vi "read_wav_to_data_fpga tester.vi"() -> ()   [LabVIEW 2021]
uses:
  <vilib>/rvi/interface/nirviOpenFPGA/nirviOpenFPGA.xnode
  <vilib>/rvi/interface/nirviReadWriteControl/nirviReadWriteControl.xnode
  <vilib>/rvi/interface/nirviMethod/nirviMethod.xnode
  <vilib>/FPGAPlugInAG/Dynamic/niLvFpga_WriteFifo_Dynamic.vi
  <vilib>/rvi/errors/niLvFpgaMergeErrorWithErrorCode.vi
  <vilib>/FPGAPlugInAG/Dynamic/niLvFpga_ReadFifo_Dynamic.vi
  <vilib>/rvi/interface/nirviCloseFPGA/nirviCloseFPGA.xnode
  <instrlib>/_niInstr/Basic Elements/v1/FPGA/niInstr Basic Elements v1 FPGA.lvlib
  <instrlib>/_niInstr/Basic Elements/v1/FPGA/Private/Count Up U16.vi
  FPGA Bitfiles/niUsrpRio200_XcvrTime.lvbitx
  chaim_vis/chaim_Tx.vi
  <vilib>/FPGAPlugInAG/USRP 294xR; 295xR 200 MSps/niLvFpga_Open_USRP 294xR; 295xR 200 MSps.vi
  <vilib>/rvi/interface/common/dynamic/niFpgaDynamicAddResources.vi
  <vilib>/FPGAPlugInAG/Dynamic/niLvFpga_ConfigureFifo_Dynamic.vi
  <vilib>/FPGAPlugInAG/Dynamic/niLvFpga_Close_Dynamic.vi
  NiFpgaLv.dll
  <vilib>/Utility/error.llb/Error Cluster From Error Code.vi
  <vilib>/rvi/interface/Simulation/niFpgaSimulationCallBeginRW.vi
  <vilib>/rvi/errors/niLvFpgaAdjustHostInterfaceError.vi
panel:
  out "Empty Elements Remaining":u32
  out "size(s)":i32
  out "wav sent out":u16
  in  "stop":bool
  in  "millisecond multiple":u32
  out "Waveform Graph 2":dbl[](graph)
  out "error out":errorcluster
  out "UP SAMPLE RATE":fxp<+,48,1>
  out "Numeric":i32
  out "Init Data Out":fxp<+/-,16,1>[](array[numeric])
  out "up sample":dbl format="%#_6f"
  out "attributes":variant
  out "Y 2":dbl[](array[numeric])
  out "dt":dbl format="%#_6p"
  out "t0":timestamp
  out "Y":dbl[](array[numeric])
  out "Waveform Graph":waveform(dbl)[](graph)
  in  "path":path
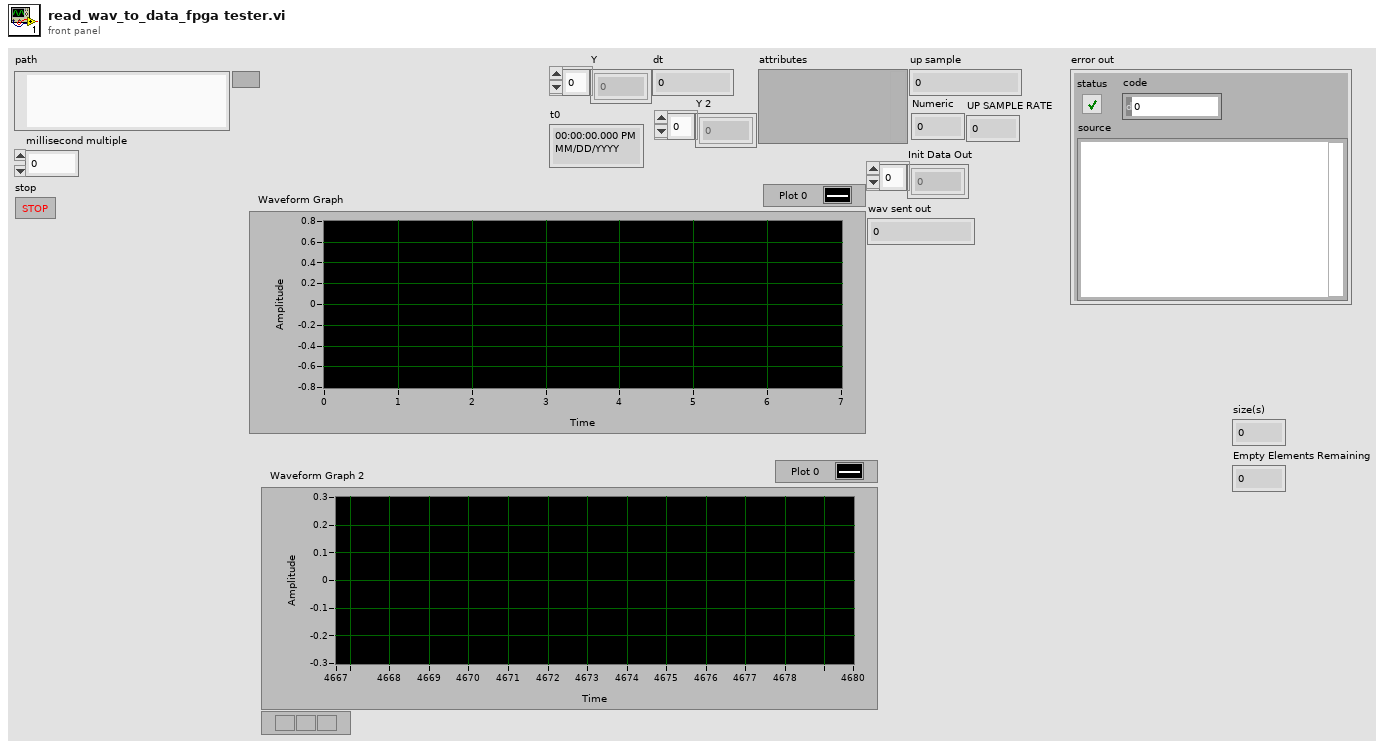
[diagram p1: front panel]
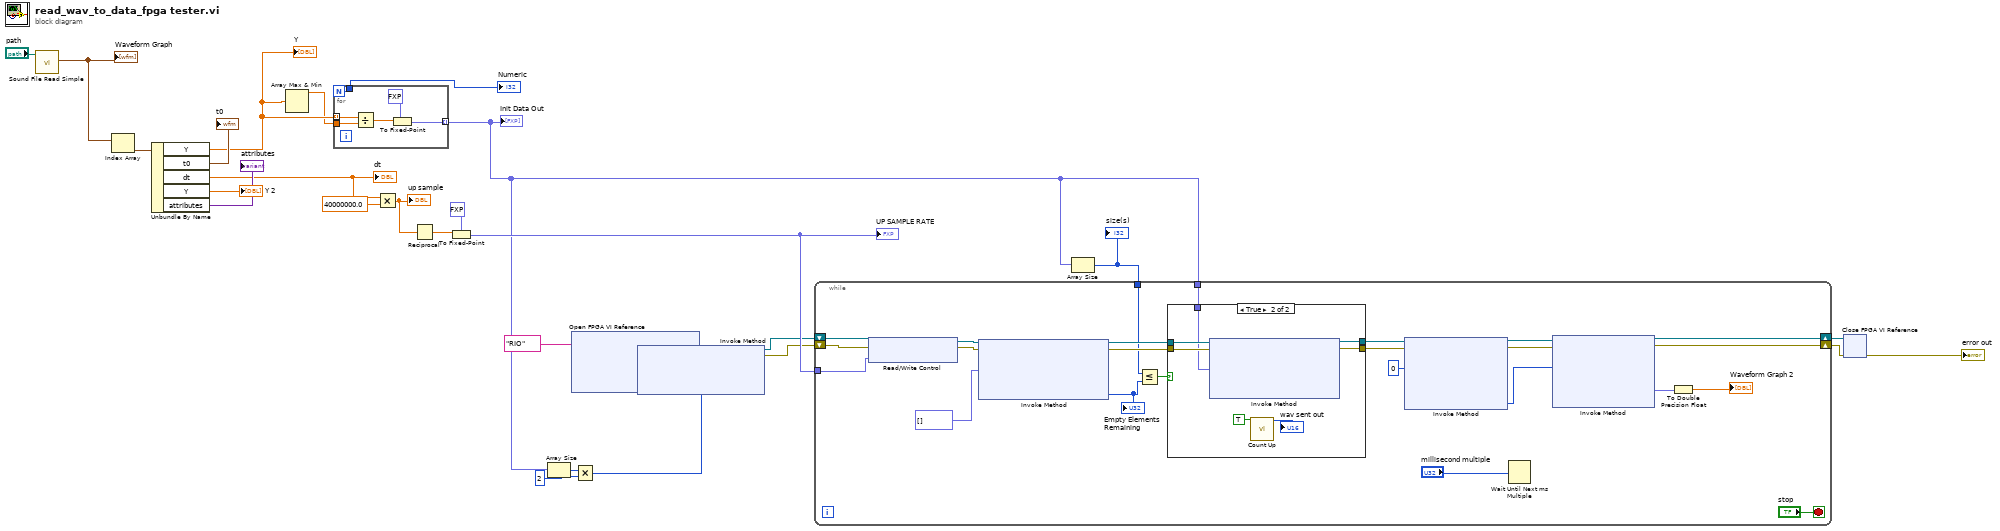
[diagram p0: block diagram]
diagram:
  n1 = call <vilib>:"Sound File Read Simple.vi"("path"="path") -> ("data"=w27:waveform(dbl)[])  [unwired: 7 in, 3 out]
  "Waveform Graph" <- w27
  n2 = Index Array(array=w27) -> (element=w26:waveform(dbl))  [unwired: 1 in]
  n3 = Unbundle By Name(w26) -> ("Y"=w20:dbl[], "t0"=→"t0":timestamp, "dt"=w22:dbl, "Y"=→"Y 2":dbl[], "attributes"=→"attributes":variant)
  "Y" <- w20
  "dt" <- w22
  n4 = Array Max & Min(array=w20) -> (max value=w19:dbl)  [unwired: 3 out]
  n5 = for {
    N -> [w29]
    tunnel: w20 -> [w34] mode=indexing
    tunnel: w19 -> [w33]
    tunnel: [w30] -> w8 mode=indexing
    tunnel: [w29] -> w18
    n6 = Divide(x=w34, y=w33) -> (x/y=w32:dbl)
    n7 = To Fixed-Point(fixed-point type=fxp<+/-,18,1> 0.0, number=w32) -> (fixed-point=w30:fxp<+/-,18,1>)
  }
  "Init Data Out" <- w8
  "Numeric" <- w18
  n8 = Multiply(x=w22, y=40000000.0) -> (x*y=w17:dbl)
  "up sample" <- w17
  n9 = Reciprocal(x=w17) -> (1/x=w16:dbl)
  n10 = To Fixed-Point(fixed-point type=fxp<+,48,1> 0.0, number=w16) -> (fixed-point=w13:fxp<+,48,1>)
  "UP SAMPLE RATE" <- w13
  n11 = Array Size(array=w8) -> (size(s)=w7:i32)
  n12 = xnode "Open FPGA VI Reference"("resource name"=tag "RIO") -> ("FPGA VI Reference Out"=w4:refnum<k20>, "error out"=w3:errorcluster)  [unwired: 1 in]
  n13 = Multiply(x=w7, y=2) -> (x*y=w5:i32)
  n14 = xnode "Invoke Method"("FPGA VI Reference In"=w4, "error in"=w3, "Requested Depth"=w5) -> ("FPGA VI Reference Out"=w2:refnum<k20>, "error out"=w1:errorcluster)  [unwired: 1 out]
  n15 = Array Size(array=w8) -> (size(s)=w12:i32)
  "size(s)" <- w12
  n16 = while {
    tunnel: w13 -> [w50]
    tunnel: w8 -> [w44]
    tunnel: w12 -> [w43]
    shift-right: [w40] -> w10
    shift-left: w2 -> [w58]
    shift-right: [w39] -> w9
    shift-left: w1 -> [w57]
    stop <- "stop" stop-if-true
    n17 = xnode "Read/Write Control"("FPGA VI Reference In"=w58, "error in"=w57, "UP SAMPLE RATE"=w50) -> ("FPGA VI Reference Out"=w49:refnum<k20>, "error out"=w46:errorcluster)
    n18 = xnode "Invoke Method"("FPGA VI Reference In"=w49, "error in"=w46, "Data"=fxp<+/-,18,1>[] []) -> ("FPGA VI Reference Out"=w48:refnum<k20>, "error out"=w47:errorcluster, "Empty Elements Remaining"=w42:u32)  [unwired: 1 in]
    "Empty Elements Remaining" <- w42
    n19 = Less Or Equal?(x=w43, y=w42) -> (x <= y?=w41:bool)
    n20 = case shown="True" w41 {
      tunnel: [w60 w67] -> w56
      tunnel: [w59 w66] -> w55
      tunnel: w48 -> [w60 w65]
      tunnel: w47 -> [w59 w64]
      tunnel: w44 -> [_ w63]
      frame False {
      }
      frame True {
        n21 = xnode "Invoke Method"("FPGA VI Reference In"=w65, "error in"=w64, "Data"=w63) -> ("FPGA VI Reference Out"=w67:refnum<k20>, "error out"=w66:errorcluster)  [unwired: 1 in, 1 out]
        n22 = call-poly <instrlib>:"Count Up.vi"("increment"=TRUE) -> ("count out"=→"wav sent out":u16)  [unwired: 14 in]
      }
    }
    n23 = xnode "Invoke Method"("FPGA VI Reference In"=w56, "error in"=w55, "Number of Elements"=u32 0) -> ("FPGA VI Reference Out"=w54:refnum<k20>, "error out"=w53:errorcluster, "Elements Remaining"=w52:u32)  [unwired: 1 in, 1 out]
    n24 = Wait Until Next ms Multiple(millisecond multiple="millisecond multiple") -> ()  [unwired: 1 out]
    n25 = xnode "Invoke Method"("FPGA VI Reference In"=w54, "error in"=w53, "Number of Elements"=w52) -> ("FPGA VI Reference Out"=w40:refnum<k20>, "error out"=w39:errorcluster, "Data"=w38:fxp<+/-,48,0>[])  [unwired: 1 in, 1 out]
    n26 = To Double Precision Float(number=w38) -> (double precision float=→"Waveform Graph 2":dbl[])
  }
  n27 = xnode "Close FPGA VI Reference"("FPGA VI Reference In"=w10, "error in"=w9) -> ("error out"=→"error out":errorcluster)
